vi "ABR-Save Data.vi"(0 "file path":path, 5 "Params":T3={"Stimulus"={"Destination"="", "Waveform"=enum."TONE PIP", "Frequency (kHz)"=16.0, "Rep rate (/sec)"=30.0, "Alternate Polarity"=FALSE, "Sampling rate (Hz)"=0.0, "Duration (ms)"=30.0, "Ramp (ms)"=5.0, "Click width (us)"=0.0, "ITI"=enum."Rate"}, "Sequence"={"Start (dB)"=25000, "Stop (dB)"=100000, "Step (dB)"=5}, "Response"={"CAP or ABR"=enum."ABR", "Gain"=10000, "Averages"=512, "Window (ms)"=8.5, "Thr Fast Steps"=8.5, "Fs (Hz)"=25000.0, "Save raw"=FALSE}, "Normalize"=FALSE, "Reject"=0.0} {"Sequence"."Start (dB)" step=5; "Response"."Thr Fast Steps" format="%.2f"; "Response"."Window (ms)" format="%.2f"; "Stimulus"."Frequency (kHz)" format="%.2f"}, 7 "StartTime":dbl, 9 "reject":dbl, 11 "error in (no error)":errorcluster, 12 "Analysis":T7, 13 "Notes":string) -> (4 "Datafile path":path, 15 "error out":errorcluster)   [LabVIEW 2020]
uses:
  Typedefs/ABR-Analysis State.ctl
  Threshold Estimation VIs/ABR3-Threshold Estimation Result.ctl
  Typedefs/ABR-Parameters.ctl
  Typedefs/ABR-Stimulus.ctl
  Typedefs/ABR-Sequence.ctl
  Typedefs/ABR-Response.ctl
  Typedefs/ABR-Data Header.ctl
  2adf8b99-1ca5-4ad6-8c2c-ba33d2e78250.vi
  epl-vi-lib/Utility VIs/Math VIs/LinSpace (x0-dx-npts).vi
  epl-vi-lib/Utility VIs/File IO VIs/Configuration File Wrapper VIs/Config-Read Key (string).vi
  CFTS VIs/CFTS-Globals.vi
panel:
  in  "STANDARD ABR":T1
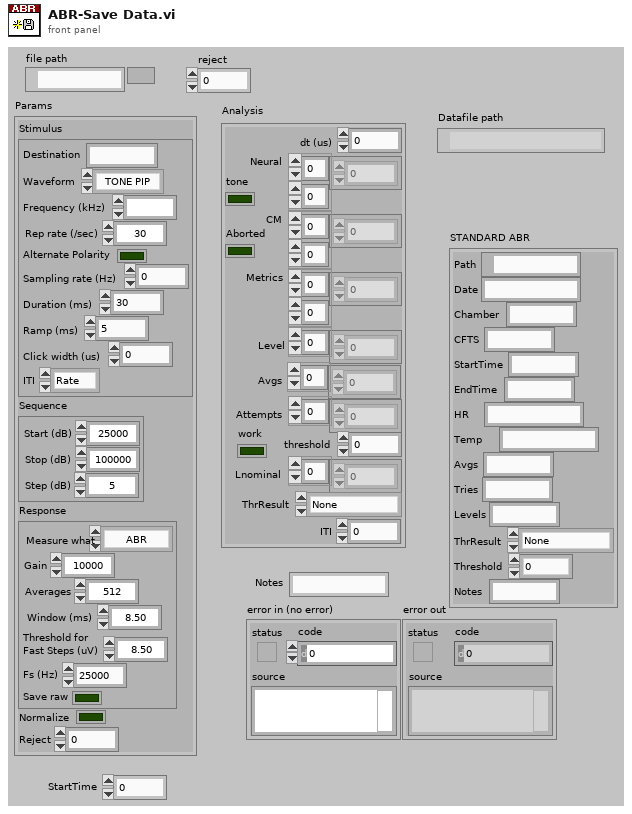
[diagram p1: front panel]
types:
  T1 = typedef "ABR-Data Header.ctl" = cluster{"Path":path, "Date":string, "Chamber":string, "CFTS":string, "StartTime":string, "EndTime":string, "HR":string, "Temp":string, "Avgs":string, "Tries":string, "Levels":string, "ThrResult":T2, "Threshold":dbl, "Notes":string}
  T2 = typedef "ABR3-Threshold Estimation Result.ctl" = enum16{"None", "Power", "Sigmoid", "Power (noisy)", "Suprathreshold", "Invalid"}
  T3 = typedef "ABR-Parameters.ctl" = cluster{"Stimulus":T4, "Sequence":T5, "Response":T6, "Normalize":bool, "Reject":dbl}
  T4 = typedef "ABR-Stimulus.ctl" = cluster{"Destination":string, "Waveform":enum16{"TONE PIP", "CLICK"}, "Frequency (kHz)":ext, "Rep rate (/sec)":dbl, "Alternate Polarity":bool, "Sampling rate (Hz)":dbl, "Duration (ms)":dbl, "Ramp (ms)":dbl, "Click width (us)":dbl, "ITI":enum16{"Rate", "Interval"}}
  T5 = typedef "ABR-Sequence.ctl" = cluster{"Start (dB)":i32, "Stop (dB)":i32, "Step (dB)":i32}
  T6 = typedef "ABR-Response.ctl" = cluster{"CAP or ABR":enum16{"CAP", "ABR"}, "Gain":i32, "Averages":i32, "Window (ms)":sgl, "Thr Fast Steps":sgl, "Fs (Hz)":dbl, "Save raw":bool}
  T7 = typedef "ABR-Analysis State.ctl" = cluster{"dt (us)":dbl, "Neural":dbl[][], "CM":dbl[][], "Metrics":dbl[][], "Level":dbl[], "Avgs":i32[], "Attempts":i32[], "Aborted":bool, "threshold":dbl, "Lnominal":dbl[], "tone":bool, "work":bool, "ThrResult":T2, "ITI":dbl}
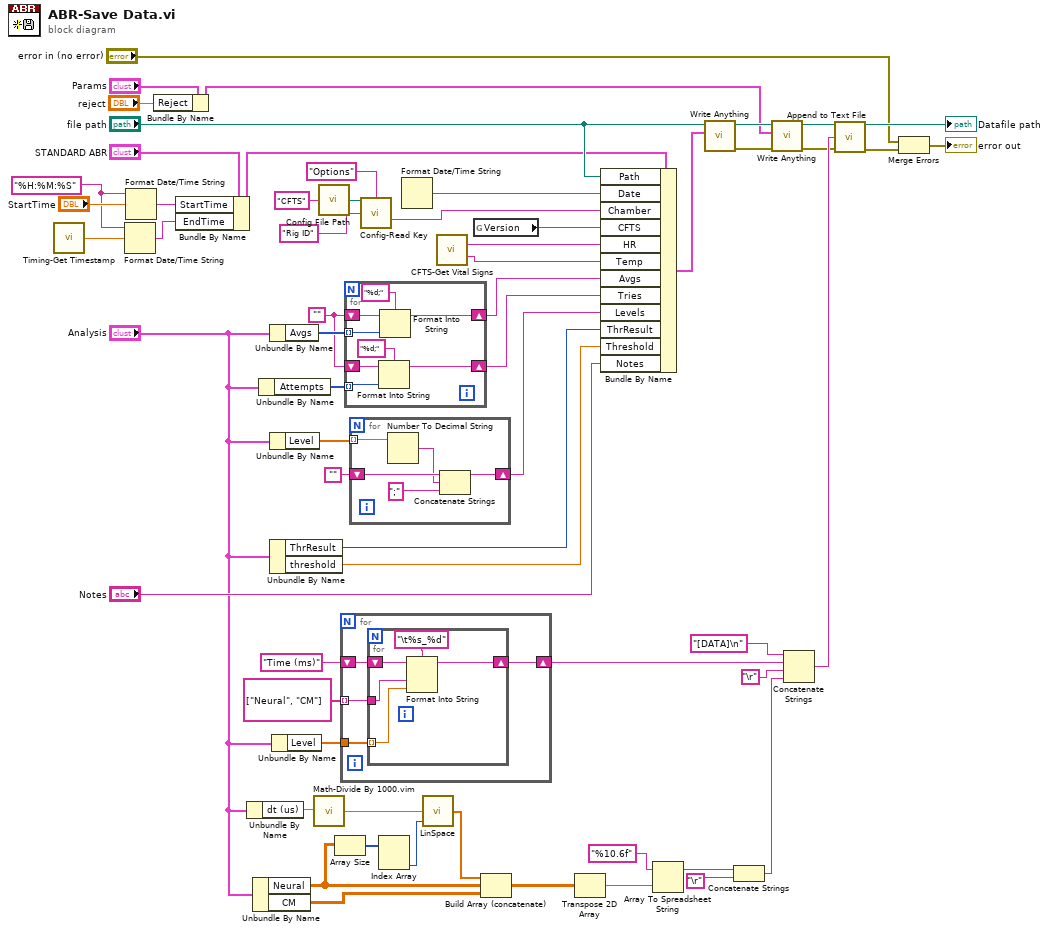
[diagram p0: block diagram]
diagram:
  w5 = "%H:%M:%S" ("time format string (%c)")
  w14 = ""
  n1 = call "Timing-Get Timestamp.vi"() -> ("double precision float"=w6:dbl)  [unwired: 14 in, 1 out]
  n2 = Format Date/Time String(time format string (%c)=w5, seconds (now)=w6) -> (date/time string=w3:string)  [unwired: 1 in]
  n3 = Format Date/Time String(time format string (%c)=w5, seconds (now)="StartTime") -> (date/time string=w4:string)  [unwired: 1 in]
  n4 = Bundle By Name(cluster="Params", "Reject"="reject") -> (w10:T3)
  n5 = Bundle By Name(cluster="STANDARD ABR", "StartTime"=w4, "EndTime"=w3) -> (w8:T1)
  n6 = Unbundle By Name("Analysis") -> ("dt (us)"=w33:dbl)
  n7 = Unbundle By Name("Analysis") -> ("Neural"=w31:dbl[][], "CM"=w48:dbl[][])
  n8 = Unbundle By Name("Analysis") -> ("Attempts"=w15:i32[])
  n9 = Unbundle By Name("Analysis") -> ("Avgs"=w16:i32[])
  n10 = Unbundle By Name("Analysis") -> ("Level"=w41:dbl[])
  n11 = Unbundle By Name("Analysis") -> ("ThrResult"=w18:T2, "threshold"=w17:dbl)
  n12 = Unbundle By Name("Analysis") -> ("Level"=w34:dbl[])
  n13 = call "Math-Divide By 1000.vim"("X"=w33) -> ("1000X"=w32:dbl)
  n14 = call "Config File Path.vi"("AppName"="CFTS") -> ("Default config file name"=w23:path)
  n15 = Array Size(array=w31) -> (size(s)=w30:i32[])
  n16 = for {
    tunnel: w34 -> [w65]
    tunnel: string[] ["Neural", "CM"] -> [w63] mode=indexing
    shift-right: [w62] -> w24
    shift-left: "Time (ms)" -> [w64]
    n17 = for {
      tunnel: w65 -> [w69] mode=indexing
      shift-right: [w67] -> w62
      shift-left: w64 -> [w68]
      tunnel: w63 -> [w66]
      n18 = Format Into String(format string="\t%s_%d", initial string=w68, w66, w69) -> (resulting string=w67:string)  [unwired: 1 in, 1 out]
    }
  }
  n19 = for {
    tunnel: w16 -> [w78] mode=indexing
    tunnel: w15 -> [w74] mode=indexing
    shift-right: [w75] -> w13
    shift-left: w14 -> [w77]
    shift-right: [w72] -> w12
    shift-left: w14 -> [w73]
    n20 = Format Into String(format string="%d;", initial string=w73, w74) -> (resulting string=w72:string)  [unwired: 1 in, 1 out]
    n21 = Format Into String(format string="%d;", initial string=w77, w78) -> (resulting string=w75:string)  [unwired: 1 in, 1 out]
  }
  n22 = for {
    shift-right: [w80] -> w40
    shift-left: "" -> [w83]
    tunnel: w41 -> [w79] mode=indexing
    n23 = Number To Decimal String(number=w79) -> (decimal integer string=w82:string)  [unwired: 1 in]
    n24 = Concatenate Strings(w83, w82, ";") -> (w80:string)
  }
  n25 = call-poly "Config-Read Key.vi"("configuration file path"=w23, "section"="Options", "key"="Rig ID" ("string")) -> ("value"=w20:string)  [unwired: 9 in, 3 out]
  n26 = Index Array(array=w30) -> (element #2=w29:i32)  [unwired: 2 in, 1 out]
  n27 = Format Date/Time String() -> (date/time string=w43:string)  [unwired: 3 in]
  n28 = call-poly "LinSpace.vi"("npts"=w29, "dx"=w32) -> ("Array"=w28:dbl[])  [unwired: 2 in, 1 out]
  n29 = call "CFTS-Get Vital Signs.vi"() -> ("HR"=w2:string, "Temp"=w1:string)  [unwired: 14 in]
  n30 = global read "CFTS-Globals.vi" "Version"() -> (w42:string)
  n31 = Build Array (concatenate)(w28, w31, w48) -> (w50:dbl[][])
  n32 = Transpose 2D Array(2D array=w50) -> (transposed array=w35:dbl[][])
  n33 = Bundle By Name(cluster=w8, "Path"="file path", "Date"=w43, "Chamber"=w20, "CFTS"=w42, "HR"=w2, "Temp"=w1, "Avgs"=w13, "Tries"=w12, "Levels"=w40, "ThrResult"=w18, "Threshold"=w17, "Notes"="Notes") -> (w46:T1)
  n34 = Array To Spreadsheet String(array=w35, 3:"%10.6f") -> (spreadsheet string=w52:string)  [unwired: 1 in]
  n35 = call "Write Anything.vi"("Anything"=w46, "Path (dialog)"="file path") -> ("Error Out"=w44:errorcluster, "Path out"=w45:path)  [unwired: 8 in]
  n36 = Concatenate Strings(w52, "\r") -> (w25:string)
  n37 = call "Write Anything.vi"("Error In"=w44, "Anything"=w10, "Path (dialog)"=w45) -> ("Error Out"=w39:errorcluster, "Path out"=w37:path)  [unwired: 7 in]
  n38 = Concatenate Strings("[DATA]\n", w24, "\r", w25) -> (w49:string)
  n39 = call "Append to Text File.vi"("file path"=w37, "text"=w49, "error in (no error)"=w39) -> ("file path out"=→"Datafile path":path, "error out"=w60:errorcluster)  [unwired: 11 in]
  n40 = Merge Errors("error in (no error)", w60) -> (→"error out":errorcluster)
